vi "DIGIT_5122_Run_Async.vi"(8 "error in (no error)":errorcluster, 10 "QMH ICR Cluster":T1, 11 "instrument handle in":refnum<k15>) -> (0 "error out":errorcluster)   [LabVIEW 2024]
doc: "This VI runs asynchronously. It starts a waveform generation in response to one or many triggers, and waits until the end of the generation before to stop."
uses:
  controls/QMH_ICR_Cluster.ctl
  controls/HARDWARE_Resources.ctl
  controls/PROCESSING_Inputs.ctl
  controls/LOOPS_Inputs.ctl
  controls/OPO_Inputs.ctl
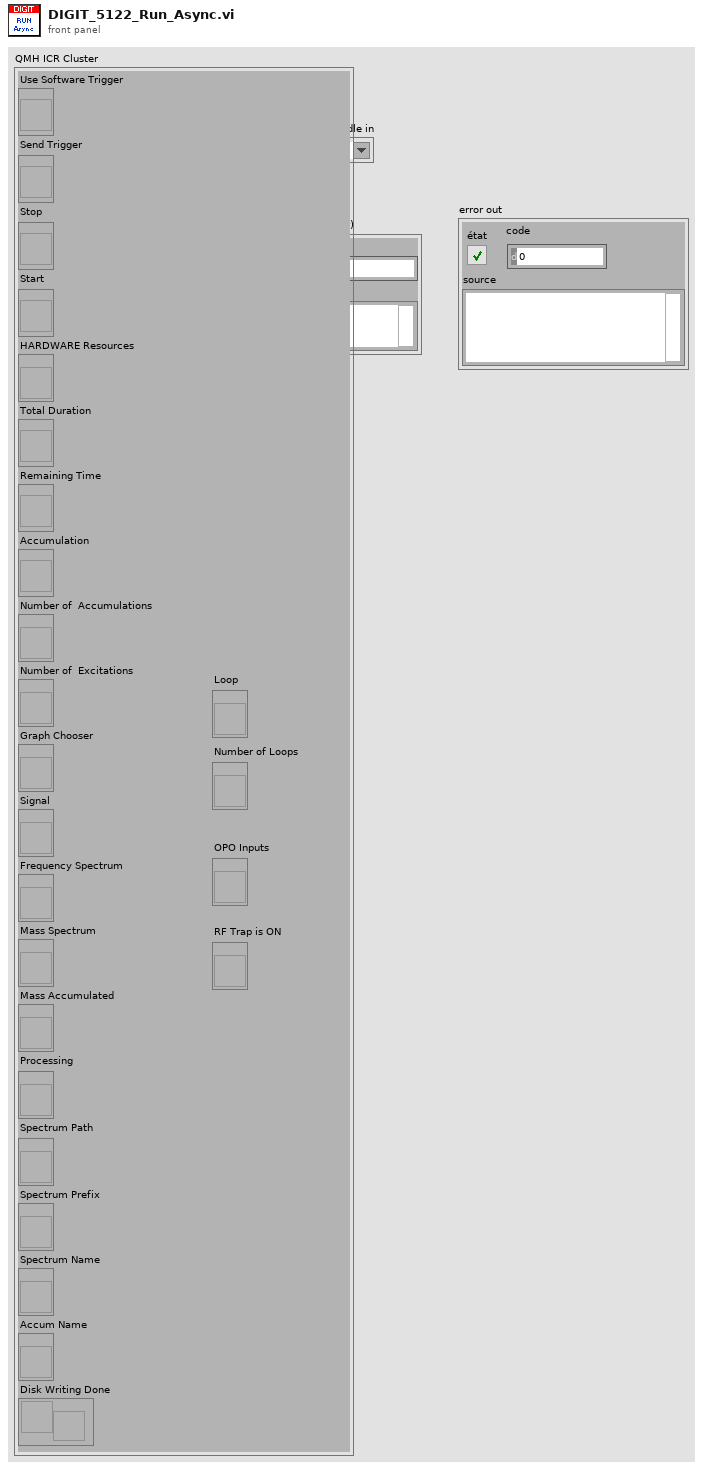
[diagram p1: front panel]
types:
  T1 = typedef "QMH_ICR_Cluster.ctl" = cluster{"Use Software Trigger":refnum<vi>, "Send Trigger":refnum<vi>, "Stop":refnum<vi>, "Start":refnum<vi>, "HARDWARE Resources":refnum<vi>, "Total Duration":refnum<vi>, "Remaining Time":refnum<vi>, "Accumulation":refnum<vi>, "Number of  Accumulations":refnum<vi>, "Number of  Excitations":refnum<vi>, "Graph Chooser":refnum<vi>, "Signal":refnum<vi>, "Frequency Spectrum":refnum<vi>, "Mass Spectrum":refnum<vi>, "Mass Accumulated":refnum<vi>, "Processing":refnum<vi>, "Spectrum Path":refnum<vi>, "Spectrum Prefix":refnum<vi>, "Spectrum Name":refnum<vi>, "Accum Name":refnum<vi>, "Disk Writing Done":refnum<notifier>, "Loop":refnum<vi>, "Number of Loops":refnum<vi>, "OPO Inputs":refnum<vi>, "RF Trap is ON":refnum<vi>}
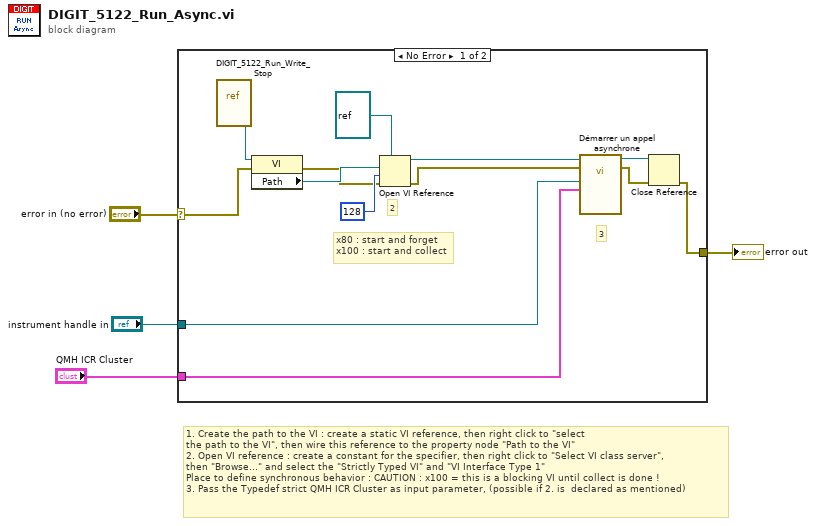
[diagram p0: block diagram]
diagram:
  # "1. Create the path to the VI : create a static VI reference, then right click to \"select\nthe path to the VI\", then wire this reference to the property node \"Path to the VI\"\n2. Open VI reference : create a constant for the specifier, then right click to \"Select VI class server\",\nthen \"Browse...\" and select the \"Strictly Typed VI\" and \"VI Interface Type 1\"\nPlace to define synchronous behavior : CAUTION : x100 = this is a blocking VI until collect is done !\n3. Pass the Typedef strict QMH ICR Cluster as input parameter, (possible if 2. is  declared as mentioned)"
  n1 = case shown="No Error" "error in (no error)" {
    selector: "error in (no error)" -> [w12 w18]
    tunnel: [w8 w18] -> w3
    tunnel: "instrument handle in" -> [w15 _]
    tunnel: "QMH ICR Cluster" -> [w6 _]
    frame No Error {
      # "3"
      # "2"
      # "x80 : start and forget\nx100 : start and collect"
      n2 = vi-ref "DIGIT_5122_Run_Write_Stop.vi"() -> (w11:refnum<vi>)
      n3 = property class="VI"(reference=w11, error in=w12) -> (error out=w13:errorcluster, "Path"=w14:path)  [unwired: 1 out]
      n4 = Open VI Reference(type specifier VI Refnum (for type only)=refnum<vi> refnum, vi path=w14, options=128, error in (no error)=w13) -> (vi reference=w5:refnum<vi>, error out=w16:errorcluster)  [unwired: 2 in]
      n5 = call-by-ref "Démarrer un appel asynchrone"(reference=w5, error in=w16, "QMH ICR Cluster"=w6, "instrument handle in"=w15) -> (reference out=w10:refnum<vi>, error out=w9:errorcluster)  [unwired: 8 in, 2 out]
      n6 = Close Reference(reference=w10, error in (no error)=w9) -> (error out=w8:errorcluster)
    }
    frame Error {
    }
  }
  "error out" <- w3
